vi "CreateSerializationSession.vi"(8 "error in":errorcluster) -> (0 "error out":errorcluster, 3 "Serialization Session ID":T1)   [LabVIEW 2019, in "grpc-lvsupport.lvlib"]
uses:
  grpc-lvsupport.lvlib
  Shared/grpcId.ctl
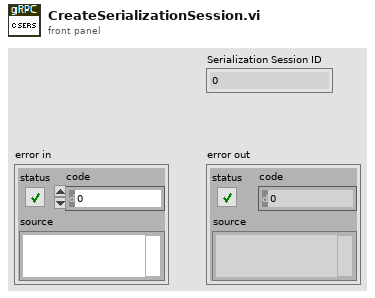
[diagram p1: front panel]
types:
  T1 = typedef "grpc-lvsupport.lvlib/grpcId.ctl" = u64
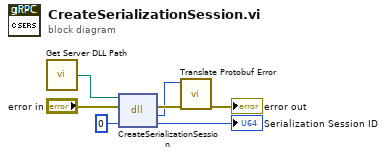
[diagram p0: block diagram]
diagram:
  n1 = call "Get Server DLL Path.vi"() -> ("Server dll path"=w5:path)
  n2 = dll-call lib="?" fn="CreateSerializationSession"(path in=w5, error in="error in", "serializationId"=u64 0 ("gRPCId")) -> (error out=w6:errorcluster, "return type"=w1:i32, "serializationId"=→"Serialization Session ID":u64)  [unwired: 1 in, 1 out]
  n3 = call "Translate Protobuf Error.vi"("error in"=w6, "Error Code"=w1) -> ("error out"=→"error out":errorcluster)  [unwired: 9 in]
